vi "temperature comparation.vi"() -> ()   [LabVIEW 2019]
uses:
  <vilib>/Instr/_visa.llb/VISA Configure Serial Port (Instr).vi
panel:
  out "Waveform Comparation":cluster{dbl, dbl, dbl}(graph) caption="Waveform Chart"
  out "?":dbl(slide) scale=0.0..100.0
  out "humidity (%)":dbl
  out "?":dbl(slide) scale=0.0..100.0
  out "?":dbl(slide) scale=0.0..100.0
  in  "stop":bool
  in  "VISA resource":refnum<visa-resource-name>
  # "Dallas"
  # "DHT22"
  # "Thermistor"
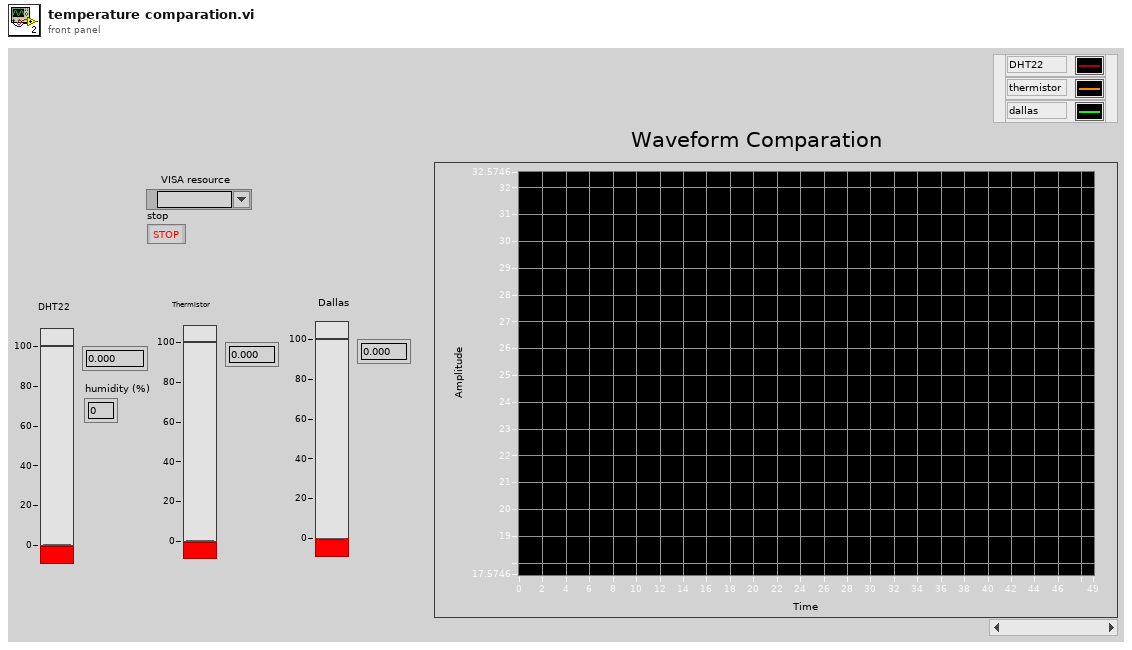
[diagram p1: front panel]
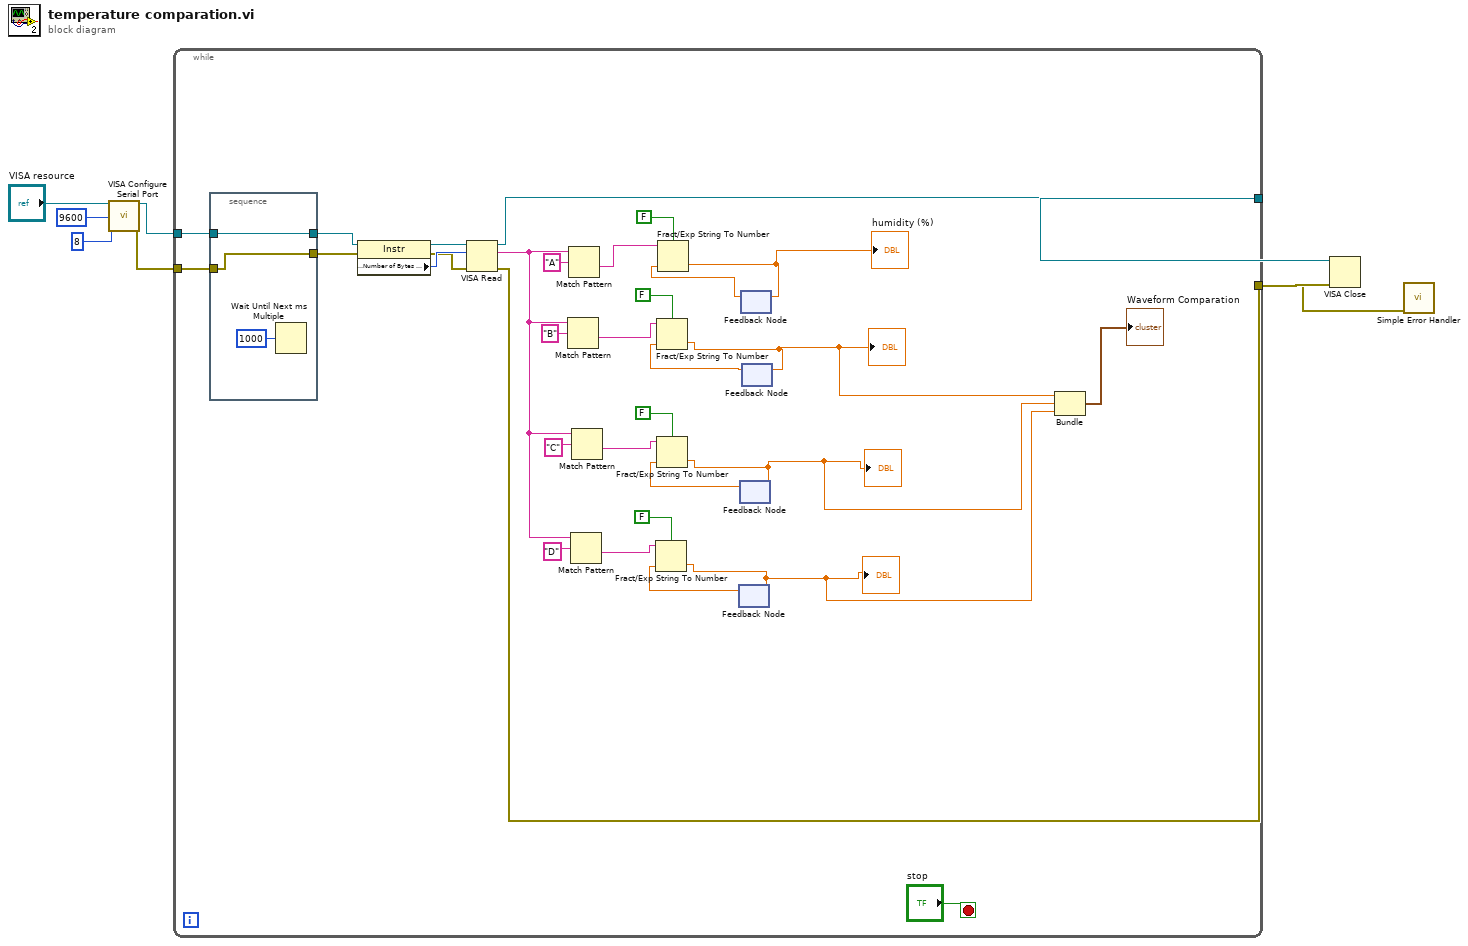
[diagram p0: block diagram]
diagram:
  n1 = call-poly "VISA Configure Serial Port"("VISA resource name"="VISA resource", "baud rate (9600)"=u32 9600, "data bits (8)"=u16 8) -> ("VISA resource name out"=w5:refnum<visa-resource-name>, "error out"=w4:errorcluster)  [unwired: 11 in]
  n2 = while {
    tunnel: w5 -> [w40]
    tunnel: w4 -> [w38]
    tunnel: [w24] -> w3
    tunnel: [w23] -> w2
    stop <- "stop" stop-if-true
    n3 = stacked-sequence {
      tunnel: w40 -> [w43]
      tunnel: [w43] -> w39
      tunnel: w38 -> [w42]
      tunnel: [w42] -> w37
      frame #0 {
        n4 = Wait Until Next ms Multiple(millisecond multiple=u32 1000) -> ()  [unwired: 1 out]
      }
    }
    n5 = property class="Instr"(reference=w39, error in=w37) -> (reference out=w36:refnum<visa-resource-name>, error out=w34:errorcluster, "Serial Settings:Number of Bytes at Serial Port"=w35:u32)
    n6 = VISA Read(VISA resource name=w36, byte count=w35, error in (no error)=w34) -> (VISA resource name out=w24:refnum<visa-resource-name>, read buffer=w14:string, error out=w23:errorcluster)  [unwired: 1 out]
    n7 = Match Pattern(string=w14, regular expression="B") -> (after substring=w29:string)  [unwired: 1 in, 3 out]
    n8 = Match Pattern(string=w14, regular expression="A") -> (after substring=w30:string)  [unwired: 1 in, 3 out]
    n9 = Match Pattern(string=w14, regular expression="D") -> (after substring=w18:string)  [unwired: 1 in, 3 out]
    n10 = Match Pattern(string=w14, regular expression="C") -> (after substring=w22:string)  [unwired: 1 in, 3 out]
    n11 = feedback #1() -> (w16:dbl)  [unwired: 1 in]
    n12 = Fract/Exp String To Number(use system decimal point (T)=FALSE, string=w18, default (0 dbl)=w16) -> (number=w10:dbl)  [unwired: 1 in, 1 out]
    "?" <- w10
    n13 = feedback-in #1(w10) -> ()
    n14 = feedback #2() -> (w20:dbl)  [unwired: 1 in]
    n15 = Fract/Exp String To Number(use system decimal point (T)=FALSE, string=w22, default (0 dbl)=w20) -> (number=w11:dbl)  [unwired: 1 in, 1 out]
    "?" <- w11
    n16 = feedback-in #2(w11) -> ()
    n17 = feedback #3() -> (w26:dbl)  [unwired: 1 in]
    n18 = Fract/Exp String To Number(use system decimal point (T)=FALSE, string=w30, default (0 dbl)=w26) -> (number=w13:dbl)  [unwired: 1 in, 1 out]
    "humidity (%)" <- w13
    n19 = feedback-in #3(w13) -> ()
    n20 = feedback #4() -> (w25:dbl)  [unwired: 1 in]
    n21 = Fract/Exp String To Number(use system decimal point (T)=FALSE, string=w29, default (0 dbl)=w25) -> (number=w12:dbl)  [unwired: 1 in, 1 out]
    "?" <- w12
    n22 = feedback-in #4(w12) -> ()
    n23 = Bundle(w12, w11, w10) -> (→"Waveform Comparation":cluster{dbl, dbl, dbl})  [unwired: 1 in]
  }
  n24 = VISA Close(VISA resource name=w3, error in (no error)=w2) -> (error out=w1:errorcluster)
  n25 = call <vilib>:"Simple Error Handler.vi"("error in (no error)"=w1) -> ()  [unwired: 4 in, 5 out]
